vi "Write Display Format.vi"(5 "Display Format":T1, 9 "Scale in":refnum<class "Scale.lvclass">) -> (3 "Scale out":refnum<class "Scale.lvclass">)   [LabVIEW 2014, in "Raspberry Pi Compatible Compiler for LabVIEW.lvlib" / "Scale.lvclass"]
uses:
  Scale.lvclass
  <vilib>/Utility/miscctls.llb/LVFormatAndPrecisionTypeDef.ctl
  Scale.lvclass/Scale.ctl
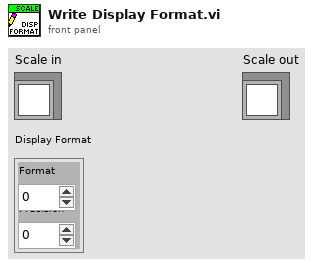
[diagram p1: front panel]
types:
  T1 = typedef "LVFormatAndPrecisionTypeDef.ctl" = cluster{"Format":u8, "Precision":u8}
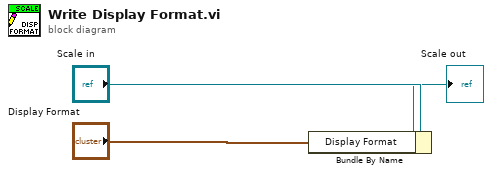
[diagram p0: block diagram]
diagram:
  n1 = Bundle By Name(cluster="Scale in", "Display Format"="Display Format") -> (→"Scale out":refnum<class "Scale.lvclass">)
